vi "SetJogConfig.vi"(8 "error in (no error)":errorcluster, 11 "KST101 in":refnum<class "KST101.lvclass">) -> (0 "error out":errorcluster, 3 "KST101 out":refnum<class "KST101.lvclass">)   [LabVIEW 2016, in "Stepper Motor Controller.lvlib" / "KST101.lvclass"]
uses:
  KST101.lvclass
  KST101.lvclass/KST101.ctl
  D:/Workspace/ProCyteOne_LaserModuleAlignment/shared/Thorlabs/Kinesis/Dependencies/Thorlabs.MotionControl.KCube.StepperMotorCLI.dll
  Dependencies/Thorlabs.MotionControl.KCube.StepperMotorCLI.dll
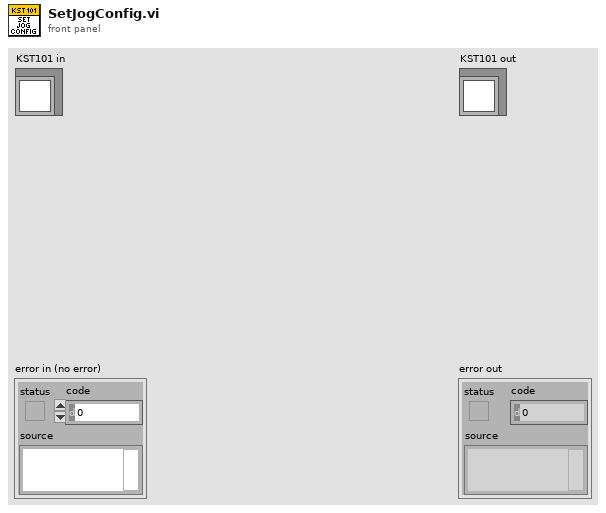
[diagram p1: front panel]
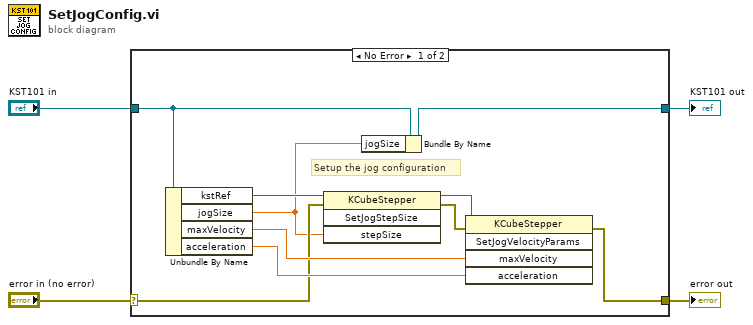
[diagram p0: block diagram]
diagram:
  n1 = case shown="No Error" "error in (no error)" {
    selector: "error in (no error)" -> [w10 w16]
    tunnel: [w9 w16] -> w3
    tunnel: [w6 w15] -> w1
    tunnel: "KST101 in" -> [w7 w15]
    frame No Error {
      # "Setup the jog configuration"
      n2 = Unbundle By Name(w7) -> ("kstRef"=w14:refnum<k24>, "jogSize"=w5:dbl, "maxVelocity"=w13:dbl, "acceleration"=w12:dbl)
      n3 = invoke class="KCubeStepper" method="SetJogStepSize"(reference=w14, error in=w10, "stepSize"=w5) -> (reference out=w8:refnum<k24>, error out=w11:errorcluster)  [unwired: 1 in, 2 out]
      n4 = Bundle By Name(cluster=w7, "jogSize"=w5) -> (w6:refnum<class "KST101.lvclass">)
      n5 = invoke class="KCubeStepper" method="SetJogVelocityParams"(reference=w8, error in=w11, "maxVelocity"=w13, "acceleration"=w12) -> (error out=w9:errorcluster)  [unwired: 1 in, 4 out]
    }
    frame Error {
    }
  }
  "error out" <- w3
  "KST101 out" <- w1
